vi "State_4ch_v00.vi"(4 "BS Hold Pulse":bool, 6 "\"I too high?\"":T6, 11 "Control Cavity Cluster":T11={"Control EPR"={"Lock"=FALSE, "Hold"=FALSE, "P Gain"=0, "P BS"=-5, "I Gain"=0, "I BS"=-10, "I2 G"=0, "I2 BS"=-26, "Scan Amp"=0, "Scan Off"=0, "Scan FS"=0, "SFS BS"=0, "I Max value"=10000, "I2 Max value"=10000, "Scope.Offset"=0, "Trigger Direction"=enum."either", "Scan-PII thresh"=0}, "Control HD A"={"Lock"=FALSE, "Hold"=FALSE, "P Gain"=0, "P BS"=-5, "I Gain"=0, "I BS"=-10, "I2 G"=0, "I2 BS"=-26, "Scan Amp"=0, "Scan Off"=0, "Scan FS"=0, "SFS BS"=0, "I Max value"=10000, "I2 Max value"=10000, "Scope.Offset"=0, "Trigger Direction"=enum."either", "Scan-PII thresh"=0}, "Control HD B"={"Lock"=FALSE, "Hold"=FALSE, "P Gain"=0, "P BS"=-5, "I Gain"=0, "I BS"=-10, "I2 G"=0, "I2 BS"=-26, "Scan Amp"=0, "Scan Off"=0, "Scan FS"=0, "SFS BS"=0, "I Max value"=10000, "I2 Max value"=10000, "Scope.Offset"=0, "Trigger Direction"=enum."either", "Scan-PII thresh"=0}, "Max"={"Max EPR"=0, "Max HD A"=0, "Max HD B"=0, "Max HD C"=0}, "Min"={"Min EPR"=0, "Min HD A"=0, "Min HD B"=0, "Min HD C"=0}, "Lock Threshold"={"EPR"=0, "HD A"=0, "HD B"=0, "HD C"=0}, "Re-Scan Threshold"={"EPR"=0, "HD A"=0, "HD B"=0, "HD C"=0}, "Lock Point?"={"EPR"=FALSE, "HD A"=FALSE, "HD B"=FALSE, "HD C"=FALSE}, "Re-scan?"={"EPR"=FALSE, "HD A"=FALSE, "HD B"=FALSE, "HD C"=FALSE}, "Lock pressed? (-1)"={"EPR"=FALSE, "HD A"=FALSE, "HD B"=FALSE, "HD C"=FALSE}, "Cavity Errors"={"EPR"=0, "HD A"=0, "HD B"=0, "HD C"=0}, "State (-1)"={"EPR"=enum."Safe", "HD A"=enum."Safe", "HD B"=enum."Safe", "HD C"=enum."Safe"}, "Safety First"={"lim reset"=FALSE, "no limit"=FALSE, "pos slew rate * dt"=0, "neg slew rate * dt"=0, "Hold All"=FALSE, "Count(Ticks)"=0}, "Control HD C"={"Lock"=FALSE, "Hold"=FALSE, "P Gain"=0, "P BS"=-5, "I Gain"=0, "I BS"=-10, "I2 G"=0, "I2 BS"=-26, "Scan Amp"=0, "Scan Off"=0, "Scan FS"=0, "SFS BS"=0, "I Max value"=10000, "I2 Max value"=10000, "Scope.Offset"=0, "Trigger Direction"=enum."either", "Scan-PII thresh"=0}}) -> (3 "PII Scan State Errors":T8={"Control EPR"={"Lock"=FALSE, "Hold"=FALSE, "P Gain"=3, "P BS"=0, "I Gain"=0, "I BS"=-10, "I2 G"=0, "I2 BS"=-26, "Scan Amp"=0, "Scan Off"=0, "Scan FS"=0, "SFS BS"=0, "I Max value"=10000, "I2 Max value"=10000, "Scope.Offset"=0, "Trigger Direction"=enum."either", "Scan-PII thresh"=0}, "Control HD A"={"Lock"=FALSE, "Hold"=FALSE, "P Gain"=0, "P BS"=-5, "I Gain"=0, "I BS"=-10, "I2 G"=0, "I2 BS"=-26, "Scan Amp"=0, "Scan Off"=0, "Scan FS"=0, "SFS BS"=0, "I Max value"=10000, "I2 Max value"=10000, "Scope.Offset"=0, "Trigger Direction"=enum."either", "Scan-PII thresh"=0}, "Control HD B"={"Lock"=FALSE, "Hold"=FALSE, "P Gain"=0, "P BS"=-5, "I Gain"=0, "I BS"=-10, "I2 G"=0, "I2 BS"=-26, "Scan Amp"=0, "Scan Off"=0, "Scan FS"=0, "SFS BS"=0, "I Max value"=10000, "I2 Max value"=10000, "Scope.Offset"=0, "Trigger Direction"=enum."either", "Scan-PII thresh"=0}, "Error Signals"={"EPR"=0, "HD A"=0, "HD B"=0, "HD C"=0}, "State"={"EPR"=enum."Safe", "HD A"=enum."Safe", "HD B"=enum."Safe", "HD C"=enum."Safe"}, "Control HD C"={"Lock"=FALSE, "Hold"=FALSE, "P Gain"=0, "P BS"=-5, "I Gain"=0, "I BS"=-10, "I2 G"=0, "I2 BS"=-26, "Scan Amp"=0, "Scan Off"=0, "Scan FS"=0, "SFS BS"=0, "I Max value"=10000, "I2 Max value"=10000, "Scope.Offset"=0, "Trigger Direction"=enum."either", "Scan-PII thresh"=0}}, 5 "MaxMin":T1)   [LabVIEW 2013]
doc: "The state of the output is decided here. There are four possible states: 1) Safe - zeros; 2) Hold - constant output of last value; 3) Scan - saw tooth at low frequency 4) Lock - PII output."
uses:
  Strict Type Defs/1BS3HD State.ctl
  Strict Type Defs/1BS3HD PII Scan State.ctl
  Strict Type Defs/PII individual.ctl
  Strict Type Defs/1BS3HD Error Signals.ctl
  Strict Type Defs/1BS3HD Lock Point.ctl
  Strict Type Defs/1BS3HD Control Cluster.ctl
  Strict Type Defs/1BS3HD Max.ctl
  Strict Type Defs/1BS3HD Min.ctl
  Strict Type Defs/1BS3HD Lock Thresh.ctl
  Strict Type Defs/Safety First.ctl
  Strict Type Defs/1BS3HD MaxMin.ctl
  Strict Type Defs/1BS3HD Reset MaxMin.ctl
panel:
  in  "MaxMin typedef":T1
  in  "Lock?":T6
  in  "PII Scan State":T8={"Control EPR"={"Lock"=FALSE, "Hold"=FALSE, "P Gain"=3, "P BS"=0, "I Gain"=0, "I BS"=-10, "I2 G"=0, "I2 BS"=-26, "Scan Amp"=0, "Scan Off"=0, "Scan FS"=0, "SFS BS"=0, "I Max value"=10000, "I2 Max value"=10000, "Scope.Offset"=0, "Trigger Direction"=enum."either", "Scan-PII thresh"=0}, "Control HD A"={"Lock"=FALSE, "Hold"=FALSE, "P Gain"=0, "P BS"=-5, "I Gain"=0, "I BS"=-10, "I2 G"=0, "I2 BS"=-26, "Scan Amp"=0, "Scan Off"=0, "Scan FS"=0, "SFS BS"=0, "I Max value"=10000, "I2 Max value"=10000, "Scope.Offset"=0, "Trigger Direction"=enum."either", "Scan-PII thresh"=0}, "Control HD B"={"Lock"=FALSE, "Hold"=FALSE, "P Gain"=0, "P BS"=-5, "I Gain"=0, "I BS"=-10, "I2 G"=0, "I2 BS"=-26, "Scan Amp"=0, "Scan Off"=0, "Scan FS"=0, "SFS BS"=0, "I Max value"=10000, "I2 Max value"=10000, "Scope.Offset"=0, "Trigger Direction"=enum."either", "Scan-PII thresh"=0}, "Error Signals"={"EPR"=0, "HD A"=0, "HD B"=0, "HD C"=0}, "State"={"EPR"=enum."Safe", "HD A"=enum."Safe", "HD B"=enum."Safe", "HD C"=enum."Safe"}, "Control HD C"={"Lock"=FALSE, "Hold"=FALSE, "P Gain"=0, "P BS"=-5, "I Gain"=0, "I BS"=-10, "I2 G"=0, "I2 BS"=-26, "Scan Amp"=0, "Scan Off"=0, "Scan FS"=0, "SFS BS"=0, "I Max value"=10000, "I2 Max value"=10000, "Scope.Offset"=0, "Trigger Direction"=enum."either", "Scan-PII thresh"=0}}
  in  "State":T2
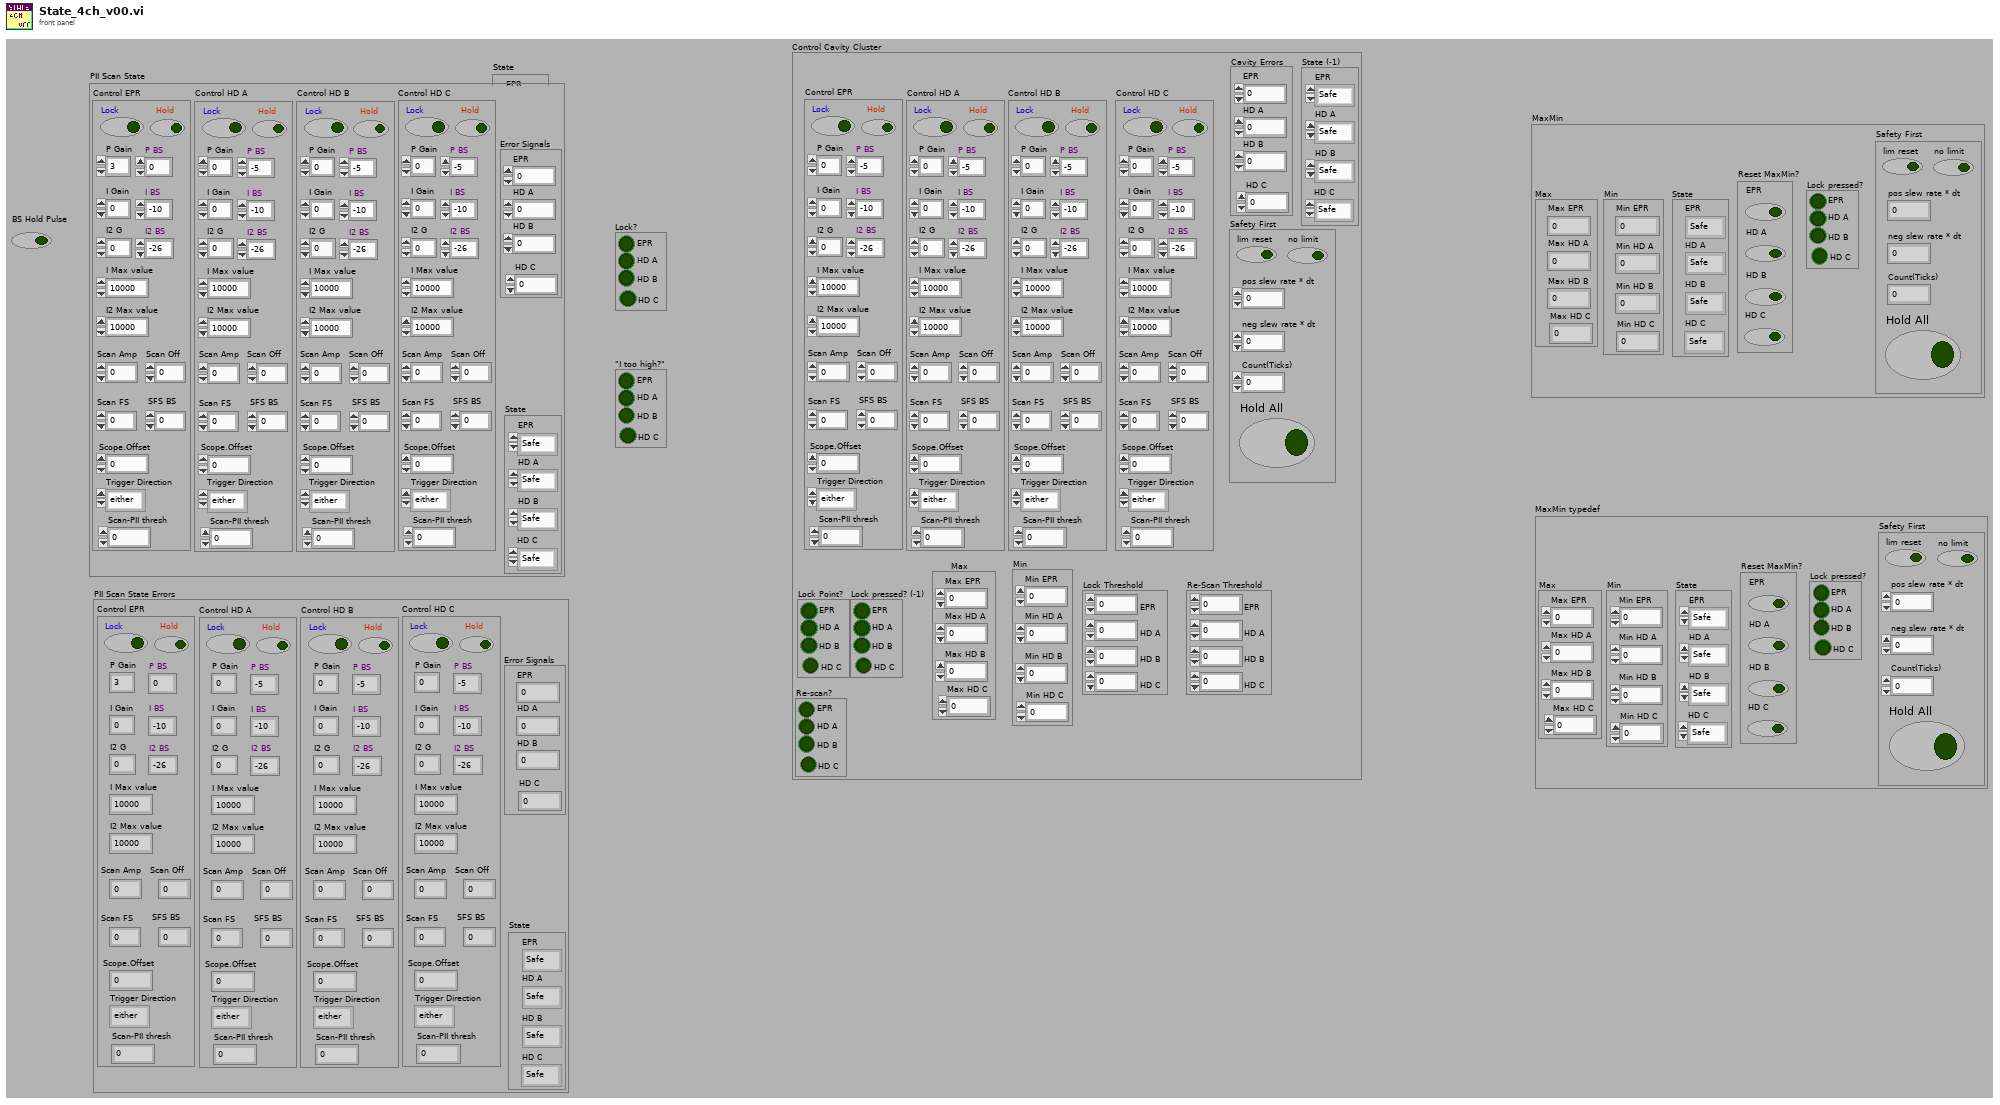
[diagram p1: front panel]
types:
  T1 = typedef "1BS3HD MaxMin.ctl" = cluster{"State":T2, "Reset MaxMin?":T3, "Max":T4, "Min":T5, "Lock pressed?":T6, "Safety First":T7}
  T2 = typedef "1BS3HD State.ctl" = cluster{"EPR":enum16{"Safe", "Hold", "Scan", "Lock"}, "HD A":enum16{"Safe", "Hold", "Scan", "Lock"}, "HD B":enum16{"Safe", "Hold", "Scan", "Lock"}, "HD C":enum16{"Safe", "Hold", "Scan", "Lock"}}
  T3 = typedef "1BS3HD Reset MaxMin.ctl" = cluster{"EPR":bool, "HD A":bool, "HD B":bool, "HD C":bool}
  T4 = typedef "1BS3HD Max.ctl" = cluster{"Max EPR":i16, "Max HD A":i16, "Max HD B":i16, "Max HD C":i16}
  T5 = typedef "1BS3HD Min.ctl" = cluster{"Min EPR":i16, "Min HD A":i16, "Min HD B":i16, "Min HD C":i16}
  T6 = typedef "1BS3HD Lock Point.ctl" = cluster{"EPR":bool, "HD A":bool, "HD B":bool, "HD C":bool}
  T7 = typedef "Safety First.ctl" = cluster{"lim reset":bool, "no limit":bool, "pos slew rate * dt":i16, "neg slew rate * dt":i16, "Hold All":bool, "Count(Ticks)":u32}
  T8 = typedef "1BS3HD PII Scan State.ctl" = cluster{"Control EPR":T9, "Control HD A":T9, "Control HD B":T9, "Error Signals":T10, "State":T2, "Control HD C":T9}
  T9 = typedef "PII individual.ctl" = cluster{"Lock":bool, "Hold":bool, "P Gain":i32, "P BS":i16, "I Gain":i32, "I BS":i16, "I2 G":i32, "I2 BS":i16, "Scan Amp":i16, "Scan Off":i16, "Scan FS":u16, "SFS BS":i16, "I Max value":i32, "I2 Max value":i32, "Scope.Offset":i16, "Trigger Direction":enum8{"either", "minus-plus", "plus-minus"}, "Scan-PII thresh":i16}
  T10 = typedef "1BS3HD Error Signals.ctl" = cluster{"EPR":i16, "HD A":i16, "HD B":i16, "HD C":i16}
  T11 = typedef "1BS3HD Control Cluster.ctl" = cluster{"Control EPR":T9, "Control HD A":T9, "Control HD B":T9, "Max":T4, "Min":T5, "Lock Threshold":T12, "Re-Scan Threshold":T12, "Lock Point?":T6, "Re-scan?":T6, "Lock pressed? (-1)":T6, "Cavity Errors":T10, "State (-1)":T2, "Safety First":T7, "Control HD C":T9}
  T12 = typedef "1BS3HD Lock Thresh.ctl" = cluster{"EPR":i16, "HD A":i16, "HD B":i16, "HD C":i16}
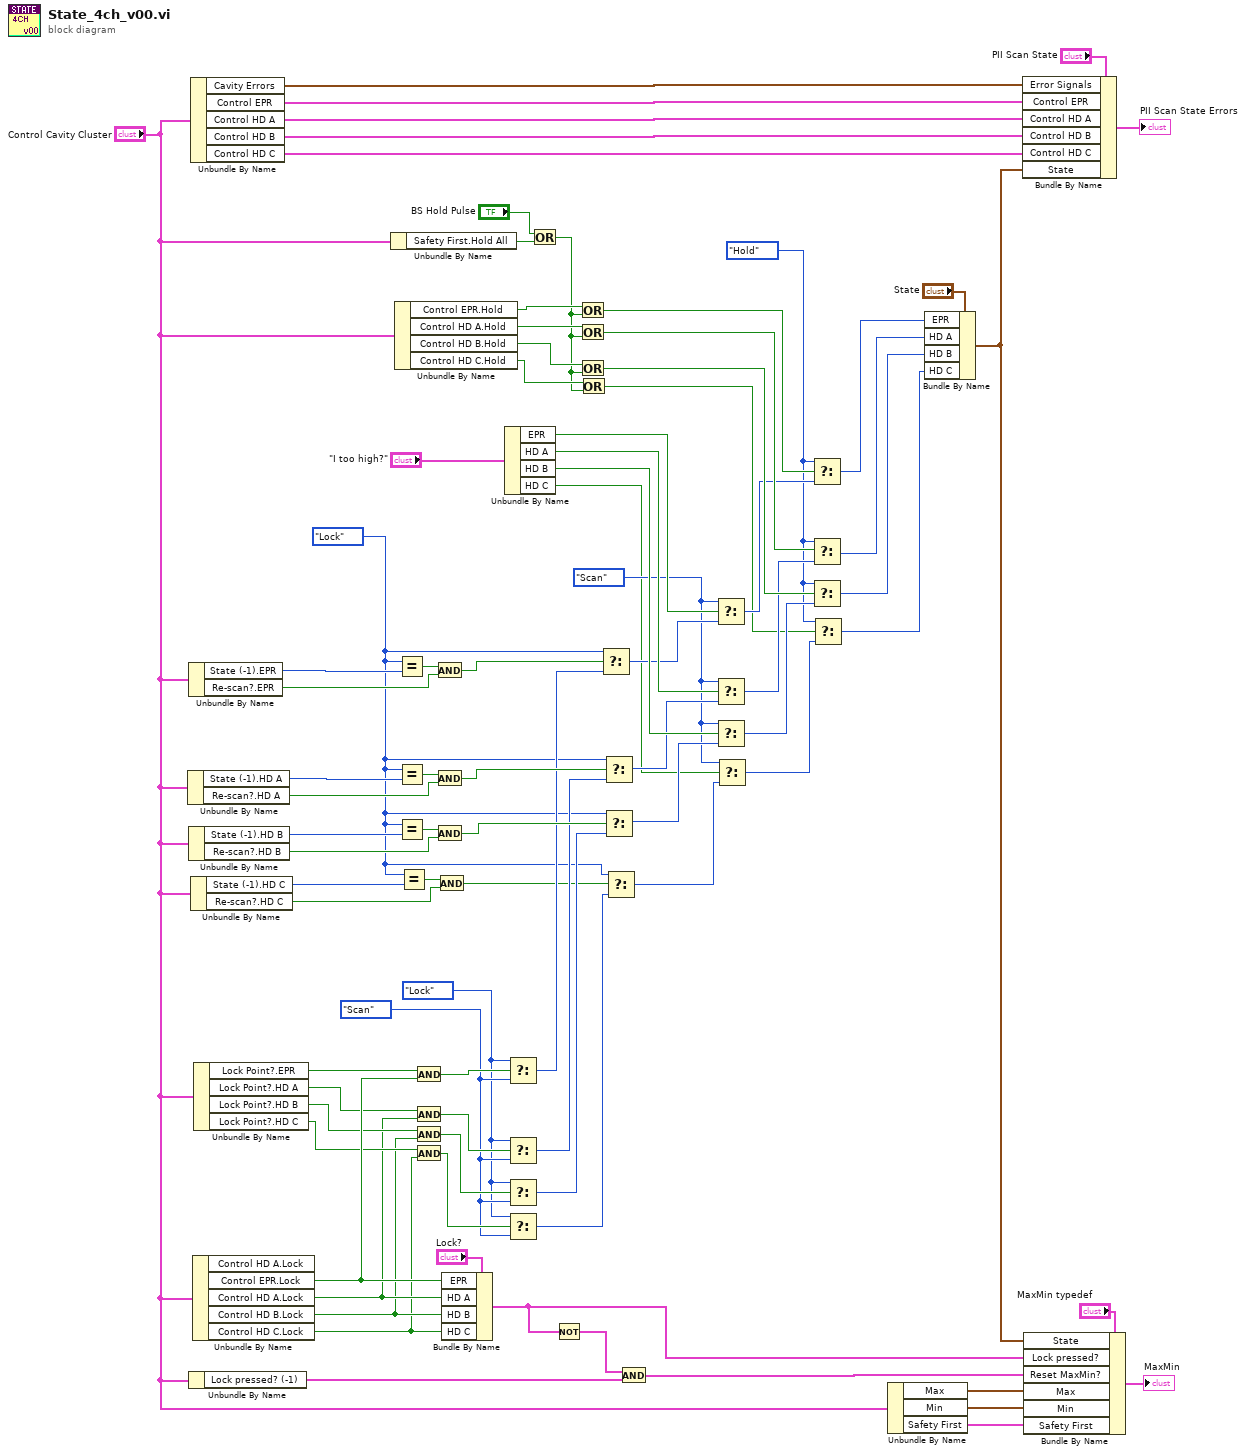
[diagram p0: block diagram]
diagram:
  w9 = enum16{"Safe", "Hold", "Scan", "Lock"}."Scan" ("State")
  w18 = enum16{"Safe", "Hold", "Scan", "Lock"}."Lock" ("y")
  w6 = enum16{"Safe", "Hold", "Scan", "Lock"}."Hold" ("State")
  w15 = enum16{"Safe", "Hold", "Scan", "Lock"}."Scan" ("State")
  w14 = enum16{"Safe", "Hold", "Scan", "Lock"}."Lock" ("State")
  n1 = Unbundle By Name("Control Cavity Cluster") -> ("State (-1).HD A"=w59:enum16{"Safe", "Hold", "Scan", "Lock"}, "Re-scan?.HD A"=w55:bool)
  n2 = Unbundle By Name("Control Cavity Cluster") -> ("State (-1).EPR"=w64:enum16{"Safe", "Hold", "Scan", "Lock"}, "Re-scan?.EPR"=w80:bool)
  n3 = Unbundle By Name("Control Cavity Cluster") -> ("State (-1).HD B"=w58:enum16{"Safe", "Hold", "Scan", "Lock"}, "Re-scan?.HD B"=w54:bool)
  n4 = Unbundle By Name("Control Cavity Cluster") -> ("Lock pressed? (-1)"=w72:T6)
  n5 = Unbundle By Name("Control Cavity Cluster") -> ("Cavity Errors"=w76:T10, "Control EPR"=w75:T9, "Control HD A"=w51:T9, "Control HD B"=w50:T9, "Control HD C"=w24:T9)
  n6 = Unbundle By Name("Control Cavity Cluster") -> ("State (-1).HD C"=w23:enum16{"Safe", "Hold", "Scan", "Lock"}, "Re-scan?.HD C"=w22:bool)
  n7 = Unbundle By Name("Control Cavity Cluster") -> ("Control EPR.Lock"=w65:bool, "Control HD A.Lock"=w12:bool, "Control HD B.Lock"=w11:bool, "Control HD C.Lock"=w1:bool)  [unwired: 1 out]
  n8 = Unbundle By Name("Control Cavity Cluster") -> ("Lock Point?.EPR"=w66:bool, "Lock Point?.HD A"=w41:bool, "Lock Point?.HD B"=w40:bool, "Lock Point?.HD C"=w17:bool)
  n9 = Unbundle By Name("Control Cavity Cluster") -> ("Safety First.Hold All"=w33:bool)
  n10 = Unbundle By Name("Control Cavity Cluster") -> ("Control EPR.Hold"=w67:bool, "Control HD A.Hold"=w49:bool, "Control HD B.Hold"=w48:bool, "Control HD C.Hold"=w4:bool)
  n11 = Equal?(x=w18, y=w64) -> (x = y?=w79:bool)
  n12 = Equal?(x=w18, y=w59) -> (x = y?=w56:bool)
  n13 = Equal?(x=w18, y=w58) -> (x = y?=w53:bool)
  n14 = Equal?(x=w18, y=w23) -> (x = y?=w21:bool)
  n15 = And(x=w66, y=w65) -> (x .and. y?=w83:bool)
  n16 = And(x=w41, y=w12) -> (x .and. y?=w47:bool)
  n17 = And(x=w40, y=w11) -> (x .and. y?=w46:bool)
  n18 = And(x=w17, y=w1) -> (x .and. y?=w16:bool)
  n19 = And(x=w79, y=w80) -> (x .and. y?=w78:bool)
  n20 = And(x=w56, y=w55) -> (x .and. y?=w57:bool)
  n21 = And(x=w53, y=w54) -> (x .and. y?=w52:bool)
  n22 = And(x=w21, y=w22) -> (x .and. y?=w19:bool)
  n23 = Bundle By Name(cluster="Lock?", "EPR"=w65, "HD A"=w12, "HD B"=w11, "HD C"=w1) -> (w61:T6)
  n24 = Unbundle By Name("\"I too high?\"") -> ("EPR"=w69:bool, "HD A"=w43:bool, "HD B"=w42:bool, "HD C"=w8:bool)
  n25 = Select(t=w14, s=w83, f=w15) -> (s? t:f=w39:enum16{"Safe", "Hold", "Scan", "Lock"})
  n26 = Select(t=w14, s=w47, f=w15) -> (s? t:f=w38:enum16{"Safe", "Hold", "Scan", "Lock"})
  n27 = Select(t=w14, s=w46, f=w15) -> (s? t:f=w37:enum16{"Safe", "Hold", "Scan", "Lock"})
  n28 = Select(t=w14, s=w16, f=w15) -> (s? t:f=w13:enum16{"Safe", "Hold", "Scan", "Lock"})
  n29 = Or(x="BS Hold Pulse", y=w33) -> (x .or. y?=w3:bool)
  n30 = Not(x=w61) -> (.not. x?=w77:T6)
  n31 = Or(x=w67, y=w3) -> (x .or. y?=w81:bool)
  n32 = Or(x=w49, y=w3) -> (x .or. y?=w45:bool)
  n33 = Or(x=w48, y=w3) -> (x .or. y?=w44:bool)
  n34 = Or(x=w4, y=w3) -> (x .or. y?=w2:bool)
  n35 = Select(t=w18, s=w78, f=w39) -> (s? t:f=w36:enum16{"Safe", "Hold", "Scan", "Lock"})
  n36 = Select(t=w18, s=w57, f=w38) -> (s? t:f=w35:enum16{"Safe", "Hold", "Scan", "Lock"})
  n37 = Select(t=w18, s=w52, f=w37) -> (s? t:f=w34:enum16{"Safe", "Hold", "Scan", "Lock"})
  n38 = Select(t=w18, s=w19, f=w13) -> (s? t:f=w10:enum16{"Safe", "Hold", "Scan", "Lock"})
  n39 = And(x=w77, y=w72) -> (x .and. y?=w70:T6)
  n40 = Select(t=w9, s=w69, f=w36) -> (s? t:f=w31:enum16{"Safe", "Hold", "Scan", "Lock"})
  n41 = Select(t=w9, s=w43, f=w35) -> (s? t:f=w30:enum16{"Safe", "Hold", "Scan", "Lock"})
  n42 = Select(t=w9, s=w42, f=w34) -> (s? t:f=w29:enum16{"Safe", "Hold", "Scan", "Lock"})
  n43 = Select(t=w9, s=w8, f=w10) -> (s? t:f=w7:enum16{"Safe", "Hold", "Scan", "Lock"})
  n44 = Select(t=w6, s=w81, f=w31) -> (s? t:f=w28:enum16{"Safe", "Hold", "Scan", "Lock"})
  n45 = Select(t=w6, s=w45, f=w30) -> (s? t:f=w27:enum16{"Safe", "Hold", "Scan", "Lock"})
  n46 = Select(t=w6, s=w44, f=w29) -> (s? t:f=w26:enum16{"Safe", "Hold", "Scan", "Lock"})
  n47 = Select(t=w6, s=w2, f=w7) -> (s? t:f=w5:enum16{"Safe", "Hold", "Scan", "Lock"})
  n48 = Unbundle By Name("Control Cavity Cluster") -> ("Max"=w63:T4, "Min"=w62:T5, "Safety First"=w60:T7)
  n49 = Bundle By Name(cluster="State", "EPR"=w28, "HD A"=w27, "HD B"=w26, "HD C"=w5) -> (w25:T2)
  n50 = Bundle By Name(cluster="PII Scan State", "Error Signals"=w76, "Control EPR"=w75, "Control HD A"=w51, "Control HD B"=w50, "Control HD C"=w24, "State"=w25) -> (→"PII Scan State Errors":T8)
  n51 = Bundle By Name(cluster="MaxMin typedef", "State"=w25, "Lock pressed?"=w61, "Reset MaxMin?"=w70, "Max"=w63, "Min"=w62, "Safety First"=w60) -> (→"MaxMin":T1)
